vi "Balance_fb.vi"(8 "error in (no error)":errorcluster, 10 "Balance":string, 11 "DB_fb_tocont in":refnum<class "DB_fb_tocont.lvclass">) -> (0 "error out":errorcluster, 3 "DB_fb_tocont out":refnum<class "DB_fb_tocont.lvclass">)   [LabVIEW 2025, in "Database_handler.lvlib" / "DB_fb_tocont.lvclass"]
uses:
  DB_fb_tocont.lvclass
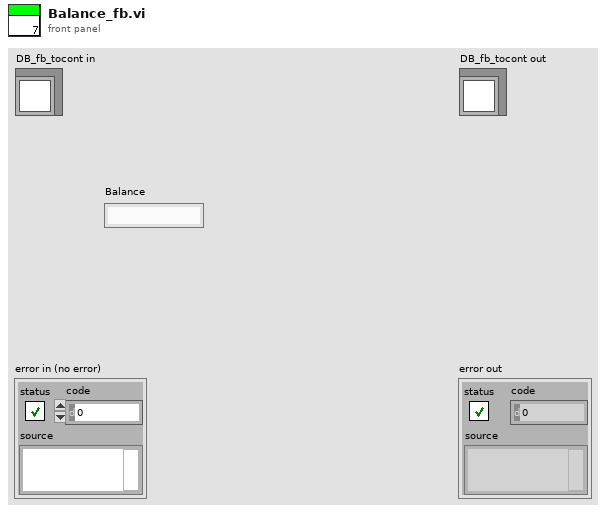
[diagram p1: front panel]
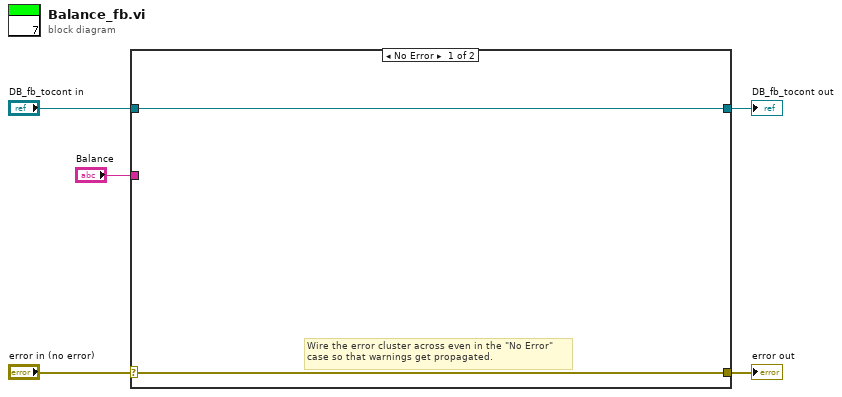
[diagram p0: block diagram]
diagram:
  n1 = case shown="No Error" "error in (no error)" {
    selector: "error in (no error)" -> [w7 w9]
    tunnel: [w7 w9] -> w4
    tunnel: [w6 w8] -> w2
    tunnel: "DB_fb_tocont in" -> [w6 w8]
    tunnel: "Balance" -> [_ _]
    frame No Error {
      # "Wire the error cluster across even in the \"No Error\"\ncase so that warnings get propagated."
    }
    frame Error {
    }
  }
  "error out" <- w4
  "DB_fb_tocont out" <- w2
